vi "Update Frame Element.vi"(9 "Detection Frame In in":T1 {"robots_blue"."height" format="%+4.3f"; "robots_blue"."pixel_y" format="%+4.3f"; "robots_blue"."pixel_x" format="%+4.3f"; "robots_blue"."orientation" format="%+4.3f"; "robots_blue"."y" format="%+4.3f"; "robots_blue"."confidence" format="%4.3f"; "robots_blue"."x" format="%+4.3f"; "robots_yellow"."height" format="%+4.3f"; "robots_yellow"."pixel_y" format="%+4.3f"; "robots_yellow"."pixel_x" format="%+4.3f"; "robots_yellow"."orientation" format="%+4.3f"; "robots_yellow"."y" format="%+4.3f"; "robots_yellow"."confidence" format="%4.3f"; "robots_yellow"."x" format="%+4.3f"}, 10 "Numeric":i32, 11 "Detection Frame In 3":T1[](array[typedef]) {"robots_blue"."height" format="%+4.3f"; "robots_blue"."pixel_y" format="%+4.3f"; "robots_blue"."pixel_x" format="%+4.3f"; "robots_blue"."orientation" format="%+4.3f"; "robots_blue"."y" format="%+4.3f"; "robots_blue"."confidence" format="%4.3f"; "robots_blue"."x" format="%+4.3f"; "robots_yellow"."height" format="%+4.3f"; "robots_yellow"."pixel_y" format="%+4.3f"; "robots_yellow"."pixel_x" format="%+4.3f"; "robots_yellow"."orientation" format="%+4.3f"; "robots_yellow"."y" format="%+4.3f"; "robots_yellow"."confidence" format="%4.3f"; "robots_yellow"."x" format="%+4.3f"}) -> (3 "Detection Frame In out":T1[](array[typedef]) {"robots_blue"."height" format="%+4.3f"; "robots_blue"."pixel_y" format="%+4.3f"; "robots_blue"."pixel_x" format="%+4.3f"; "robots_blue"."orientation" format="%+4.3f"; "robots_blue"."y" format="%+4.3f"; "robots_blue"."confidence" format="%4.3f"; "robots_blue"."x" format="%+4.3f"; "robots_yellow"."height" format="%+4.3f"; "robots_yellow"."pixel_y" format="%+4.3f"; "robots_yellow"."pixel_x" format="%+4.3f"; "robots_yellow"."orientation" format="%+4.3f"; "robots_yellow"."y" format="%+4.3f"; "robots_yellow"."confidence" format="%4.3f"; "robots_yellow"."x" format="%+4.3f"})   [LabVIEW 2017]
uses:
  SSL Detection Robot.ctl
  SSL Detection Ball.ctl
  SSL Detection Frame.ctl
  <vilib>/Analysis/Matrix/Datatypes/RealMatrix.ctl
  <vilib>/Analysis/Matrix/NI_Matrix.lvlib
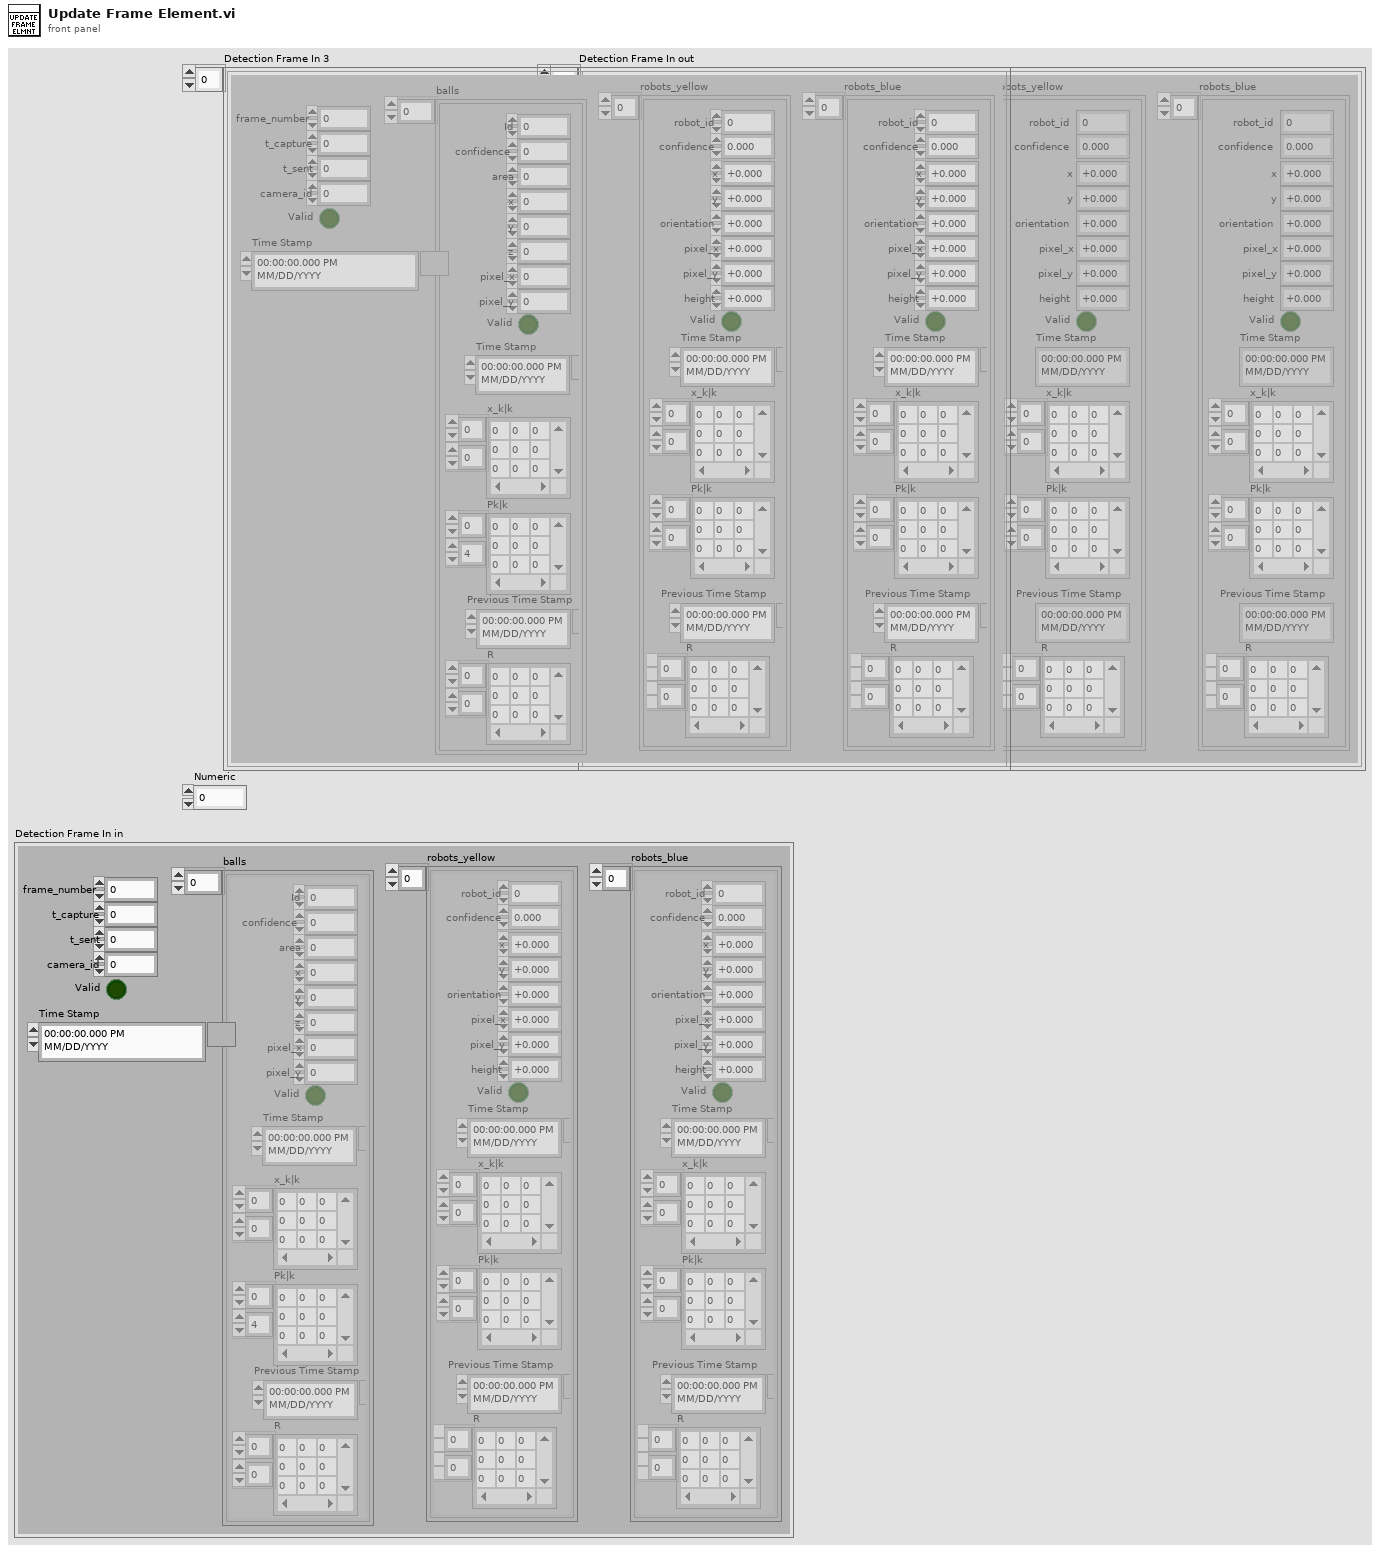
[diagram p1: front panel]
types:
  T1 = typedef "SSL Detection Frame.ctl" = cluster{"frame_number":u32, "t_capture":dbl, "t_sent":dbl, "camera_id":u32, "robots_yellow":T2[], "robots_blue":T2[], "balls":T4[], "Valid":bool, "Time Stamp":timestamp}
  T2 = typedef "SSL Detection Robot.ctl" = cluster{"x":sgl, "robot_id":u32, "confidence":sgl, "y":sgl, "orientation":sgl, "pixel_x":sgl, "pixel_y":sgl, "height":sgl, "Valid":bool, "Time Stamp":timestamp, "x_k|k":T3, "Pk|k":T3, "Previous Time Stamp":timestamp, "R":T3}
  T3 = typedef "NI_Matrix.lvlib/RealMatrix.ctl" = dbl[][]
  T4 = typedef "SSL Detection Ball.ctl" = cluster{"x":sgl, "area":u32, "confidence":sgl, "y":sgl, "z":sgl, "pixel_x":sgl, "pixel_y":sgl, "Valid":bool, "Time Stamp":timestamp, "x_k|k":T3, "Pk|k":T3, "Id":u32, "Previous Time Stamp":timestamp, "R":T3}
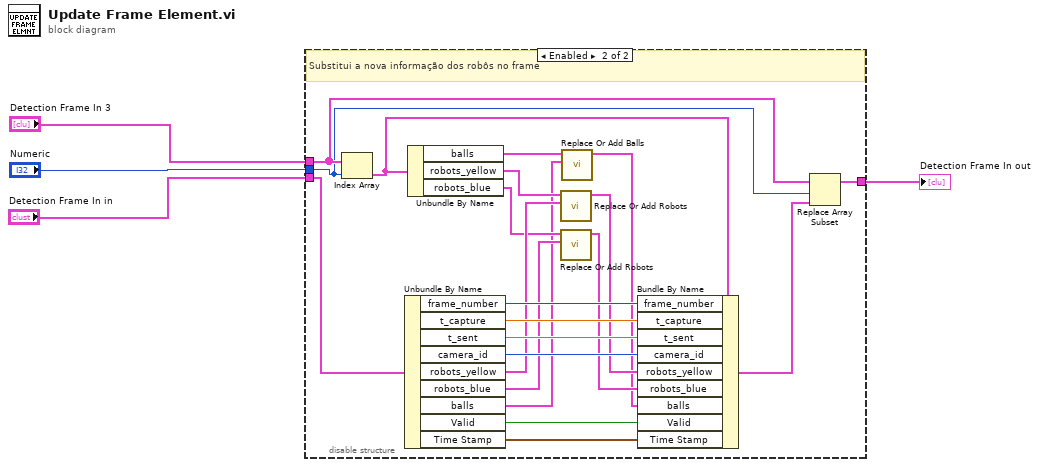
[diagram p0: block diagram]
diagram:
  n1 = disable-structure shown="Enabled" {
    disable-tunnel: "Detection Frame In 3" -> [_ w11]
    disable-tunnel: "Numeric" -> [_ w9]
    disable-tunnel: "Detection Frame In in" -> [_ w24]
    disable-tunnel: [_ w8] -> w4
    frame Disabled {
    }
    frame Enabled {
      # "Substitui a nova informação dos robôs no frame"
      n2 = Index Array(array=w11, index=w9) -> (element=w25:T1)
      n3 = Unbundle By Name(w24) -> ("frame_number"=w23:u32, "t_capture"=w22:dbl, "t_sent"=w21:dbl, "camera_id"=w20:u32, "robots_yellow"=w16:T2[], "robots_blue"=w13:T2[], "balls"=w6:T4[], "Valid"=w19:bool, "Time Stamp"=w18:timestamp)
      n4 = Unbundle By Name(w25) -> ("balls"=w7:T4[], "robots_yellow"=w17:T2[], "robots_blue"=w14:T2[])
      n5 = call "Replace Or Add Robots.vi"("Robots New"=w16, "Robots Old"=w17) -> ("Robots New Out"=w15:T2[])  [unwired: 9 in]
      n6 = call "Replace Or Add Robots.vi"("Robots New"=w13, "Robots Old"=w14) -> ("Robots New Out"=w12:T2[])  [unwired: 9 in]
      n7 = call "Replace Or Add Balls.vi"("balls new"=w6, "balls"=w7) -> ("Balls out"=w5:T4[])  [unwired: 9 in]
      n8 = Bundle By Name(cluster=w25, "frame_number"=w23, "t_capture"=w22, "t_sent"=w21, "camera_id"=w20, "robots_yellow"=w15, "robots_blue"=w12, "balls"=w5, "Valid"=w19, "Time Stamp"=w18) -> (w10:T1)
      n9 = Replace Array Subset(array=w11, new element=w10, index=w9) -> (w8:T1[])
    }
  }
  "Detection Frame In out" <- w4
